vi "Report.vi"(8 "error in":errorcluster, 9 "Received":path, 10 "Approved":path, 11 "Report With WinMerge in":refnum<class "Report With WinMerge.lvclass">) -> (0 "error out":errorcluster, 2 "Worked?":bool, 3 "Report With WinMerge out":refnum<class "Report With WinMerge.lvclass">)   [LabVIEW 2020, in "Approval Tests.lvlib" / "Report With WinMerge.lvclass"]
uses:
  Report With WinMerge.lvclass
  Approval Tests.lvlib
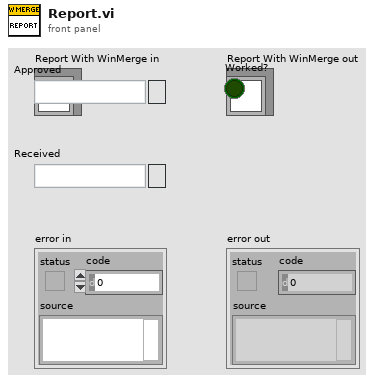
[diagram p1: front panel]
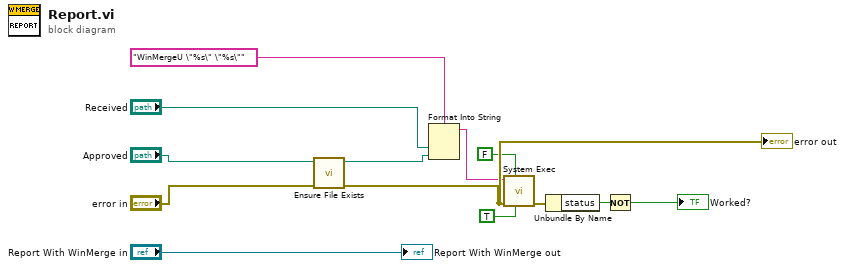
[diagram p0: block diagram]
diagram:
  n1 = call "Ensure File Exists.vi"("error in"="error in", "Approved"="Approved") -> ("error out"=w11:errorcluster, "File Path"=w1:path)  [unwired: 8 in]
  "error out" <- w11
  n2 = Format Into String(format string="WinMergeU \"%s\" \"%s\"", "Received", w1) -> (resulting string=w8:string)  [unwired: 2 in, 1 out]
  n3 = call <vilib>:"System Exec.vi"("run minimized? (F)"=TRUE, "wait until completion? (T)"=FALSE, "error in (no error)"=w11, "command line"=w8) -> ("error out"=w13:errorcluster)  [unwired: 4 in, 3 out]
  n4 = Unbundle By Name(w13) -> ("status"=w4:bool)
  n5 = Not(x=w4) -> (.not. x?=→"Worked?":bool)
  "Report With WinMerge out" <- "Report With WinMerge in"
